vi "Timed Progress-Bar.vi"(0 "Delay Label":string, 1 "Size":dbl, 2 "Increment":dbl) -> (6 "Prog Bar Ref":refnum<vi>)   [LabVIEW 2018]
panel:
  out "Slide":i32(slide) scale=0.0..100.0
  # "%"
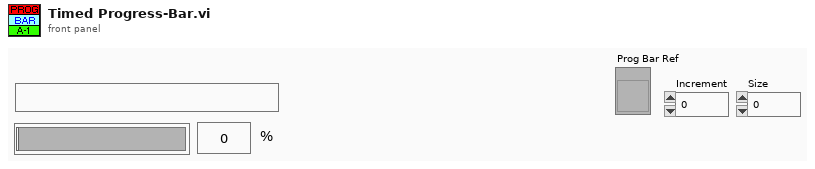
[diagram p1: front panel]
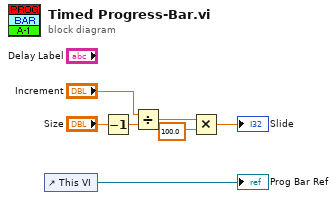
[diagram p0: block diagram]
diagram:
  n1 = control-ref of="This VI"() -> (→"Prog Bar Ref":refnum<vi>)
  n2 = Decrement(x="Size") -> (x-1=w4:dbl)
  n3 = Divide(x="Increment", y=w4) -> (x/y=w3:dbl)
  n4 = Multiply(x=w3, y=100.0) -> (x*y=→"Slide":dbl)
